vi "Sensors.vi"(11 "Ultrasonic Sensor":T1) -> ()   [LabVIEW 2013]
uses:
  <vilib>/Rock Robotics/WPI/AnalogChannel/WPI_AnalogChannelDevRef.ctl
  <vilib>/Rock Robotics/SystemInterfaces/Typedef/FPGA_TypedefAnalogModule.ctl
  <vilib>/Rock Robotics/SystemInterfaces/AI/FPGA_AIChannel.ctl
  Events.vi
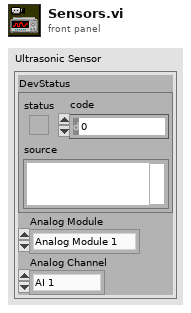
[diagram p1: front panel]
types:
  T1 = typedef "WPI_AnalogChannelDevRef.ctl" = cluster{"DevStatus":errorcluster, "Analog Module":T2, "Analog Channel":T3}
  T2 = typedef "FPGA_TypedefAnalogModule.ctl" = enum16{"Analog Module 1", "Analog Module 2"}
  T3 = typedef "FPGA_AIChannel.ctl" = enum8{"AI 1", "AI 2", "AI 3", "AI 4", "AI 5", "AI 6", "AI 7", "AI 8", "Invalid"}
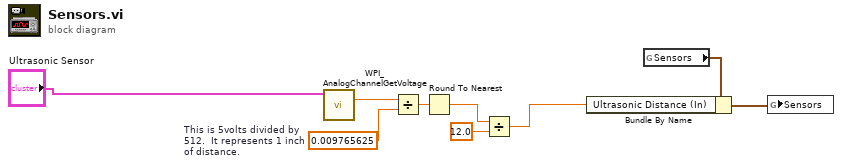
[diagram p0: block diagram]
diagram:
  w6 = 0.009765625  # This is 5volts divided by 512.  It represents 1 inch of distance.
  n1 = call <vilib>:"WPI_AnalogChannelGetVoltage.vi"("AIDeviceRef"="Ultrasonic Sensor") -> ("Voltage"=w7:dbl)  [unwired: 8 in, 2 out]
  n2 = Divide(x=w7, y=w6) -> (x/y=w5:dbl)
  n3 = Round To Nearest(number=w5) -> (nearest integer value=w3:dbl)
  n4 = Divide(x=w3, y=12.0) -> (x/y=w2:dbl)
  n5 = global read "Events.vi" "Sensors"() -> (w8:cluster{"Ultrasonic Distance (In)":dbl})
  n6 = Bundle By Name(cluster=w8, "Ultrasonic Distance (In)"=w2) -> (w9:cluster{"Ultrasonic Distance (In)":dbl})
  n7 = global write "Events.vi" "Sensors"(w9) -> ()
